vi "Global_GameOver.vi"() -> ()   [LabVIEW 2018]
panel:
  out "GameOver":bool
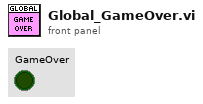
[diagram p1: front panel]
diagram:
